vi "Find Tension.vi"(11 "Desired Tension":dbl) -> (2 "At Tension?":bool, 3 "Motor Output":dbl)   [LabVIEW 2013]
uses:
  <vilib>/addons/control/pid/pid.llb/PID Control Input Filter (DBL).vi
  <vilib>/addons/control/pid/pid.llb/PID (DBL).vi
  <vilib>/addons/control/pid/NI_PID_pid.lvlib
panel:
  in  "Tension overcome coefficient":dbl
  out "Tension":dbl
  in  "Threshold":dbl=0.04
  out "Filtered":dbl(graph)
  out "Target":dbl(graph)
  in  "PID gains":T1={"proportional gain (Kc)"=4.5, "integral time (Ti, min)"=0.01, "derivative time (Td, min)"=1.0} {"derivative time (Td, min)" format="%.3f"; "integral time (Ti, min)" format="%.3f"; "proportional gain (Kc)" format="%.3f"}
  in  "output range":cluster{"output high":dbl, "output low":dbl}={"output high"=1.0, "output low"=-1.0} {"output low" format="%.2f"; "output high" format="%.2f"}
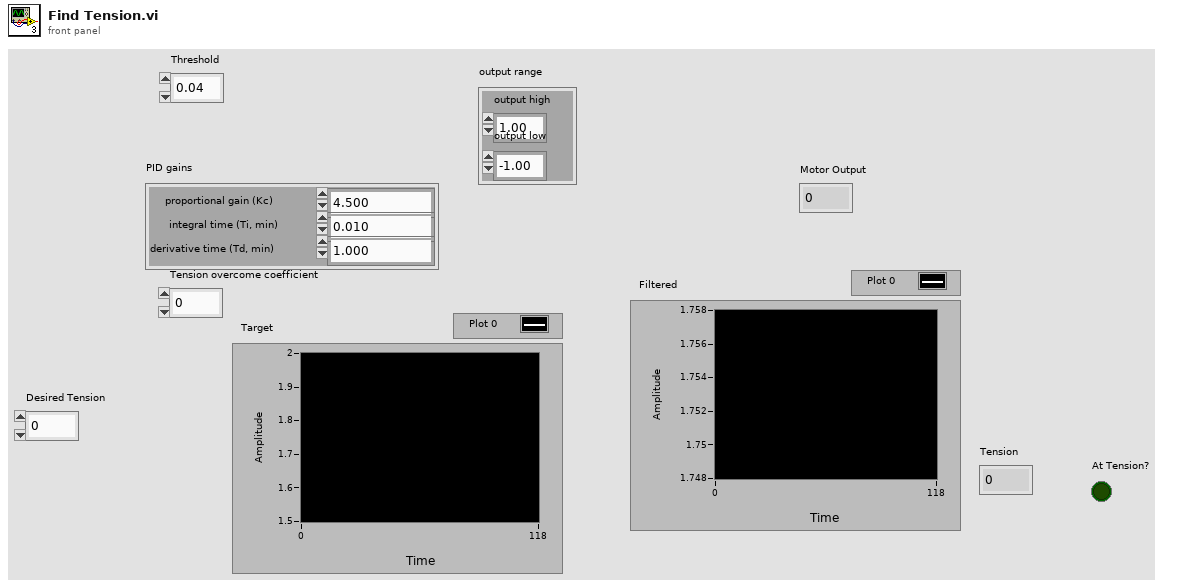
[diagram p1: front panel]
types:
  T1 = cluster{"proportional gain (Kc)":dbl, "integral time (Ti, min)":dbl, "derivative time (Td, min)":dbl}
  T2 = typedef "WPI_AnalogChannelDevRef.ctl" = cluster{"DevStatus":errorcluster, "Analog Module":T3, "Analog Channel":T4}
  T3 = typedef "FPGA_TypedefAnalogModule.ctl" = enum16{"Analog Module 1", "Analog Module 2"}
  T4 = typedef "FPGA_AIChannel.ctl" = enum8{"AI 1", "AI 2", "AI 3", "AI 4", "AI 5", "AI 6", "AI 7", "AI 8", "Invalid"}
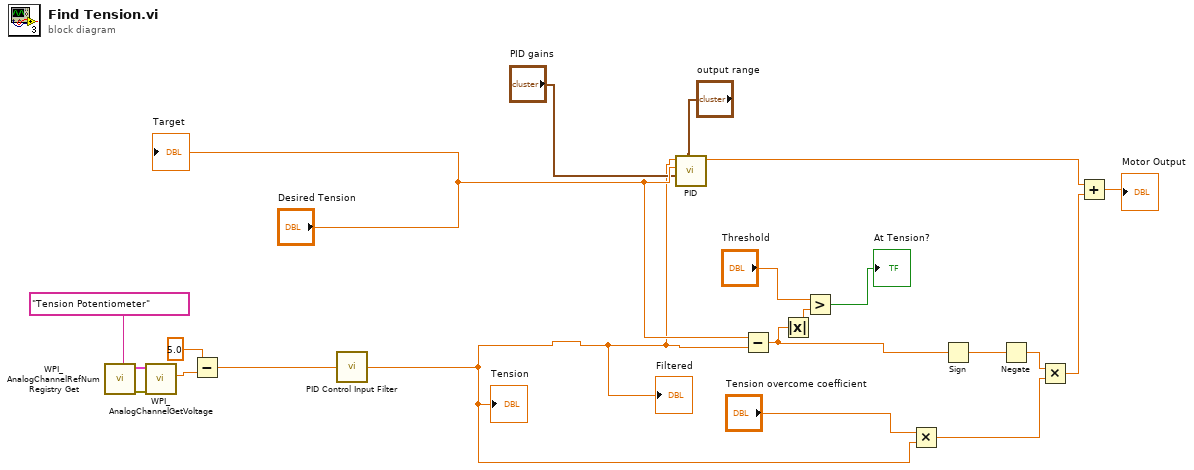
[diagram p0: block diagram]
diagram:
  n1 = call <vilib>:"WPI_AnalogChannelRefNum Registry Get.vi"("refnum name"="Tension Potentiometer") -> ("error out"=w21:errorcluster, "AIDeviceRef"=w20:T2)  [unwired: 9 in]
  n2 = call <vilib>:"WPI_AnalogChannelGetVoltage.vi"("error in (no error)"=w21, "AIDeviceRef"=w20) -> ("Voltage"=w18:dbl)  [unwired: 7 in, 2 out]
  n3 = Subtract(x=5.0, y=w18) -> (x-y=w3:dbl)
  n4 = call-poly <vilib>:"PID Control Input Filter.vi"("input"=w3) -> ("output"=w4:dbl)  [unwired: 4 in]
  "Filtered" <- w4
  "Tension" <- w4
  n5 = call-poly <vilib>:"PID.vi"("output range"="output range", "PID gains"="PID gains", "process variable"="Desired Tension", "setpoint"=w4) -> ("output"=w5:dbl)  [unwired: 6 in, 1 out]
  n6 = Subtract(x="Desired Tension", y=w4) -> (x-y=w9:dbl)
  n7 = Absolute Value(x=w9) -> (abs(x)=w10:dbl)
  n8 = Greater?(x="Threshold", y=w10) -> (0:→"At Tension?":bool)
  n9 = Multiply(x="Tension overcome coefficient", y=w4) -> (x*y=w8:dbl)
  n10 = Sign(1:w9) -> (0:w2:dbl)
  n11 = Negate(x=w2) -> (-x=w1:dbl)
  n12 = Multiply(x=w1, y=w8) -> (x*y=w6:dbl)
  n13 = Add(x=w5, y=w6) -> (x+y=→"Motor Output":dbl)
  "Target" <- "Desired Tension"
